vi "WaitForAcquisitionUpdate.vi"(5 "ReadoutTimeout":i32, 8 "error in":errorcluster, 9 "frame size (bytes)":i32, 10 "readout_stride (bytes)":i32, 11 "camera handler in":u64) -> (0 "error out":errorcluster, 1 "Status":T1, 2 "read_count * frames":u16[][](array[numeric]), 3 "camera handler out":u64)   [LabVIEW 2014, in "PICam.lvlib"]
doc: "Picam_GetCameraID() returns the ID associates with a specified camera handle."
uses:
  PICam.lvlib
  Picam32.dll
panel:
  out "Errors_out":u32
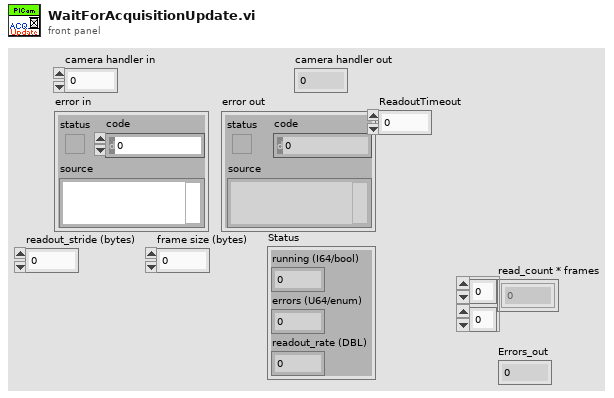
[diagram p1: front panel]
types:
  T1 = cluster{"running (I64/bool)":i32, "errors (U64/enum)":u32, "readout_rate (DBL)":dbl}
  T2 = cluster{"running (I32/bool)":i32, "errors (U32/enum)":u32, "readout_rate (DBL)":dbl}
  T3 = cluster{"initial_readout*":u64, "readout_count":i64}
  T4 = cluster{"initial_readout*":u32, "dummy filler":u32, "readout_count":i64}
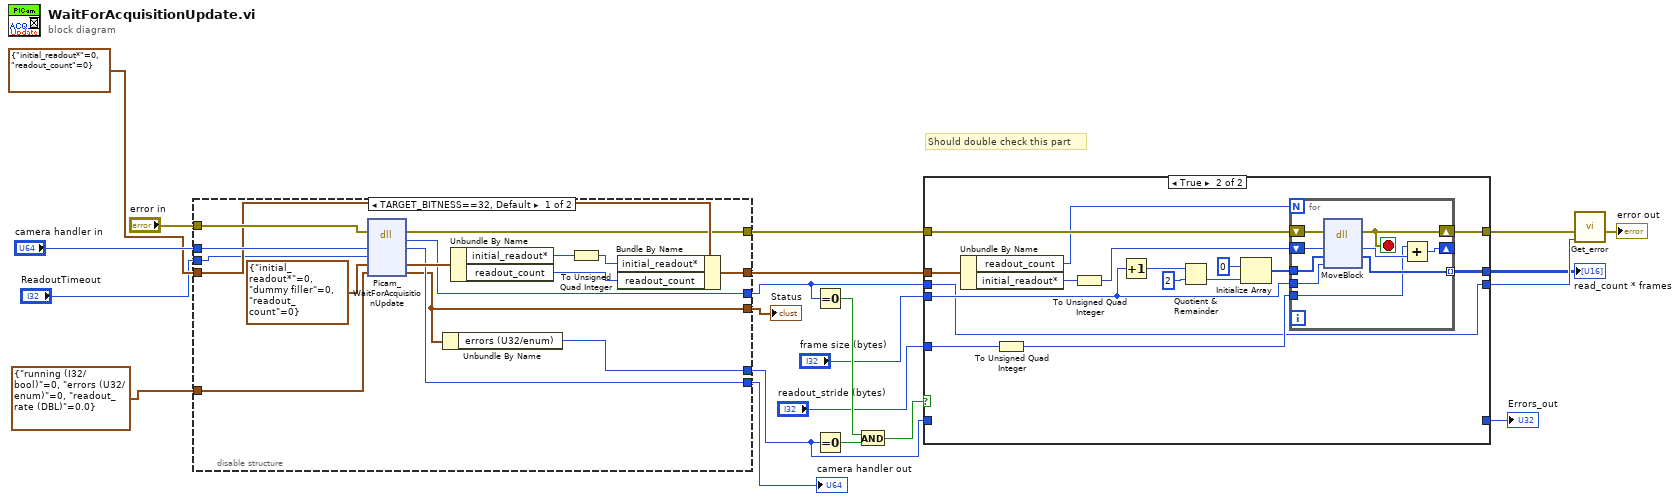
[diagram p0: block diagram]
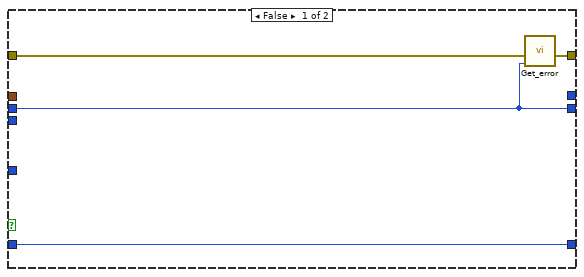
[diagram p2: hidden frame]
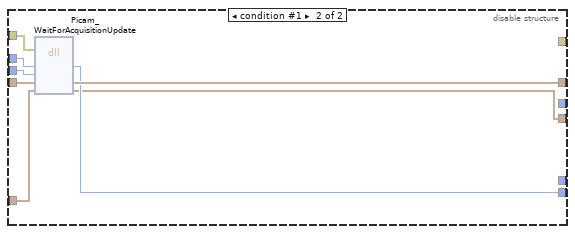
[diagram p3: hidden frame]
diagram:
  # "Should double check this part"
  n1 = disable-structure shown="TARGET_BITNESS==32, Default" {
    disable-tunnel: "camera handler in" -> [w37 w45]
    disable-tunnel: "error in" -> [w36 w44]
    disable-tunnel: T3 {"initial_readout*"=0, "readout_count"=0} -> [w31 w43]
    disable-tunnel: [w29 w42] -> w3
    disable-tunnel: [w28 w40] -> w18
    disable-tunnel: [w27 _] -> w9
    disable-tunnel: [w26 _] -> w8
    disable-tunnel: [w24 w39] -> w16
    disable-tunnel: "ReadoutTimeout" -> [w25 w41]
    disable-tunnel: [w23 _] -> w2
    disable-tunnel: T2 {"running (I32/bool)"=0, "errors (U32/enum)"=0, "readout_rate (DBL)"=0.0} -> [w22 w38]
    frame condition #0 (active) {
      n2 = dll-call lib="Picam32.dll" fn="Picam_WaitForAcquisitionUpdate"(error in=w36, "camera_handle"=w37, "ReadoutTimeout"=w25, "availableData"=T4 {"initial_readout*"=0, "dummy filler"=0, "readout_count"=0}, "status"=w22) -> (error out=w27:errorcluster, "return type"=w26:i32, "camera_handle"=w28:u64, "availableData"=w32:T4, "status"=w24:T2)  [unwired: 3 in, 1 out]
      n3 = Unbundle By Name(w24) -> ("errors (U32/enum)"=w23:u32)
      n4 = Unbundle By Name(w32) -> ("initial_readout*"=w34:u32, "readout_count"=w33:i64)
      n5 = To Unsigned Quad Integer(1:w34) -> (0:w30:u64)
      n6 = Bundle By Name(cluster=w31, "initial_readout*"=w30, "readout_count"=w33) -> (w29:T3)
    }
    frame condition #1 {
      n7 = dll-call lib="Picam32.dll" fn="Picam_WaitForAcquisitionUpdate"(error in=w44, "camera_handle"=w45, "ReadoutTimeout"=w41, "availableData"=w43, w38) -> ("camera_handle"=w40:u64, "availableData"=w42:T3, w39:T2)  [unwired: 4 in, 2 out]
    }
  }
  "camera handler out" <- w18
  "Status" <- w16
  n8 = Equal To 0?(x=w8) -> (x = 0?=w14:bool)
  n9 = Equal To 0?(x=w2) -> (x = 0?=w13:bool)
  n10 = And(x=w14, y=w13) -> (x .and. y?=w12:bool)
  n11 = case shown="True" w12 {
    tunnel: w9 -> [w49 w65]
    tunnel: w8 -> [w46 w51]
    tunnel: w2 -> [w47 _]
    tunnel: w3 -> [_ w50]
    tunnel: "readout_stride (bytes)" -> [_ w62]
    tunnel: "frame size (bytes)" -> [_ w56]
    tunnel: [_ w54] -> w5
    tunnel: [w48 w52] -> w6
    tunnel: [w47 _] -> w4
    tunnel: [w46 w51] -> w7
    frame False {
      n12 = call "Get_error.vi"("PICam_Error"=w46, "error in (no error)"=w49) -> ("error out"=w48:errorcluster)  [unwired: 9 in]
    }
    frame True {
      n13 = Unbundle By Name(w50) -> ("readout_count"=w64:i64, "initial_readout*"=w63:u64)
      n14 = To Unsigned Quad Integer(1:w62) -> (0:w61:u64)
      n15 = To Unsigned Quad Integer(1:w63) -> (0:w53:u64)
      n16 = Increment(x=w56) -> (x+1=w59:i32)
      n17 = Quotient & Remainder(x=w59, y=2) -> (floor(x/y)=w57:i32)  [unwired: 1 out]
      n18 = Initialize Array(u16 0 ("element"), w57) -> (w55:u16[])
      n19 = for {
        N: w64 -> [_]
        shift-right: [w73] -> w52
        shift-left: w65 -> [w74]
        shift-right: [w71] -> _
        shift-left: w53 -> [w72]
        tunnel: w61 -> [w66]
        tunnel: w56 -> [w70]
        tunnel: w55 -> [w69]
        tunnel: [w68] -> w54 mode=indexing
        stop <- w73 stop-if-true
        n20 = dll-call lib="LabVIEW" fn="MoveBlock"(error in=w74, "src"=w72, "tgt"=w69, "size"=w70) -> (error out=w73:errorcluster, "src"=w67:u64, "tgt"=w68:u16[])  [unwired: 4 in, 1 out]
        n21 = Add(x=w66, y=w67) -> (x+y=w71:u64)
      }
    }
  }
  "Errors_out" <- w4
  "read_count * frames" <- w5
  n22 = call "Get_error.vi"("PICam_Error"=w7, "error in (no error)"=w6) -> ("error out"=→"error out":errorcluster)  [unwired: 9 in]
